vi "Random.vi"() -> ()   [LabVIEW 2013]
panel:
  in  "Number of Points":i32
  out "Waveform Chart":dbl[](graph)
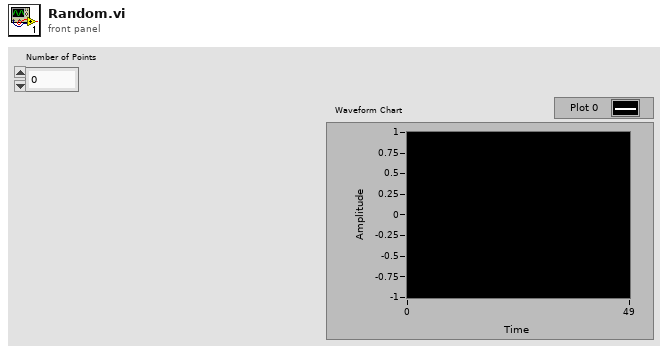
[diagram p1: front panel]
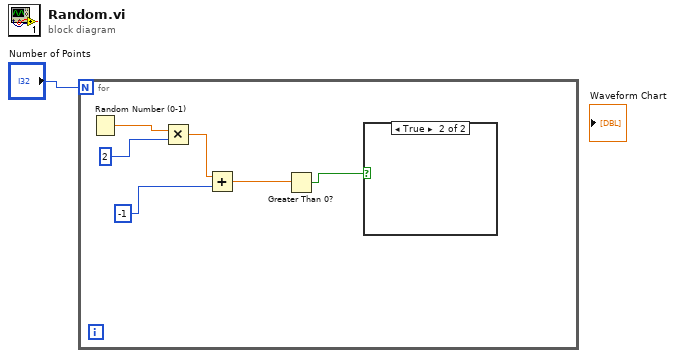
[diagram p0: block diagram]
diagram:
  n1 = for {
    N: "Number of Points" -> [_]
    n2 = Random Number (0-1)() -> (number: 0 to 1=w7:dbl)
    n3 = Multiply(x=w7, y=2) -> (x*y=w5:dbl)
    n4 = Add(x=w5, y=-1) -> (x+y=w3:dbl)
    n5 = Greater Than 0?(x=w3) -> (x > 0?=w2:bool)
    n6 = case shown="True" w2 {
      frame False {
      }
      frame True {
      }
    }
  }
